vi "Find All Clusters.vi"(8 "Error In":errorcluster, 11 "VI In":refnum<vi>) -> (0 "Error Out":errorcluster, 2 "Clusters":refnum<vi>[](array[refnum]), 3 "VI Out":refnum<vi>)   [LabVIEW 2018, in "Toolkit.lvlib"]
doc: "Finds all cluster constants and controls in a VI. Cluster constants only appear on the Block Diagram while cluster controls are only recognized as clusters on the Front Panel. Cluster controls only appear as a generic terminal on the Block Diagram. Thus, this VI finds all clusters on the Block Diagram and all clusters on the Front Panel."
uses:
  Toolkit.lvlib
  <vilib>/Utility/traverseref.llb/TRef TravTarget.ctl
  <vilib>/Utility/traverseref.llb/VI Scripting - Traverse.lvlib
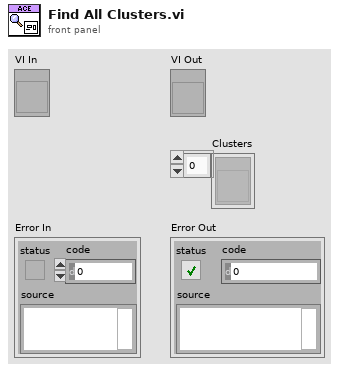
[diagram p1: front panel]
types:
  T1 = typedef "TRef TravTarget.ctl" = enum16{"FP", "BD", "Other"}
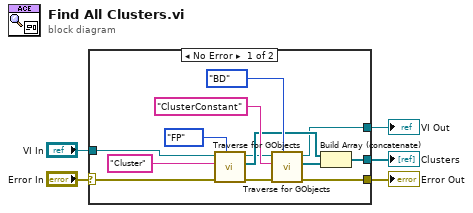
[diagram p0: block diagram]
diagram:
  n1 = case shown="No Error" "Error In" {
    selector: "Error In" -> [w18 w19]
    tunnel: "VI In" -> [w10 w20]
    tunnel: [w8 w20] -> w3
    tunnel: [w7 w19] -> w2
    tunnel: [w6 _] -> w1
    frame No Error {
      n2 = call <vilib>:"Traverse for GObjects.vi"("Traverse Target"=TRef_TravTarget."FP", "error in (no error)"=w18, "Class Name"="Cluster", "VI Refnum"=w10) -> ("error out"=w13:errorcluster, "References"=w12:refnum<vi>[], "dup VI Refnum"=w9:refnum<vi>)  [unwired: 4 in, 1 out]
      n3 = call <vilib>:"Traverse for GObjects.vi"("Traverse Target"=TRef_TravTarget."BD", "error in (no error)"=w13, "Class Name"="ClusterConstant", "VI Refnum"=w9) -> ("error out"=w7:errorcluster, "References"=w11:refnum<vi>[], "dup VI Refnum"=w8:refnum<vi>)  [unwired: 4 in, 1 out]
      n4 = Build Array (concatenate)(w12, w11) -> (w6:refnum<vi>[])
    }
    frame Error {
    }
  }
  "VI Out" <- w3
  "Error Out" <- w2
  "Clusters" <- w1
